vi "DiableEnumItems.vi"(7 "Number Of Channels":i32=8, 11 "Enum in":refnum<vi>) -> ()   [LabVIEW 2013]
uses:
  <vilib>/Analysis/1siggen.llb/Ramp Pattern by Delta.vi
  <vilib>/Analysis/NI_AALBase.lvlib
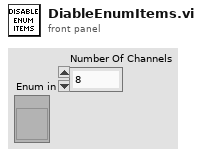
[diagram p1: front panel]
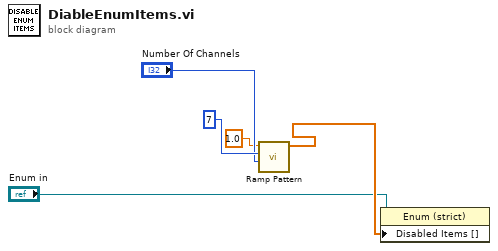
[diagram p0: block diagram]
diagram:
  n1 = call-poly <vilib>:"Ramp Pattern.vi"("start"="Number Of Channels", "end"=7 ("x"), "delta"=1.0) -> ("Ramp Pattern"=w3:dbl[])  [unwired: 6 in, 2 out]
  n2 = property class="Enum (strict)"(reference="Enum in", "Disabled Items []"=w3) -> ()  [unwired: 1 in, 2 out]
